vi "write_data.vi"(8 "error in (no error)":errorcluster, 10 "data":T1, 11 "IsotonicRegression in":refnum<class "IsotonicRegression.lvclass">) -> (0 "error out":errorcluster, 3 "IsotonicRegression out":refnum<class "IsotonicRegression.lvclass">)   [LabVIEW 2020, in "IsotonicRegression.lvclass"]
uses:
  IsotonicRegression.lvclass
  Controls/isotonic_regression_data.ctl
  IsotonicRegression.lvclass/IsotonicRegression.ctl
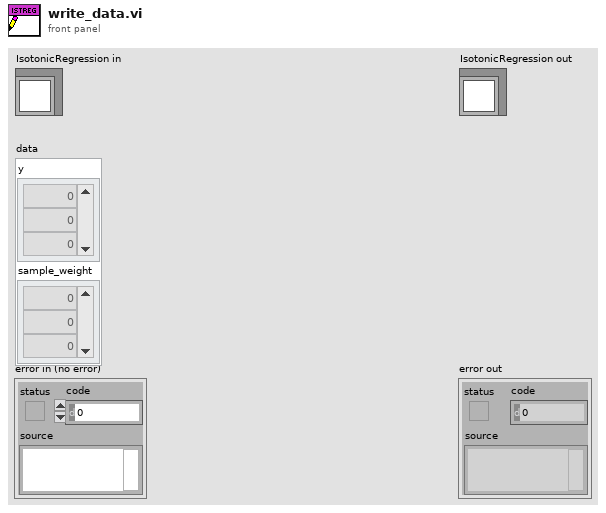
[diagram p1: front panel]
types:
  T1 = typedef "isotonic_regression_data.ctl" = cluster{"y":dbl[], "sample_weight":dbl[]}
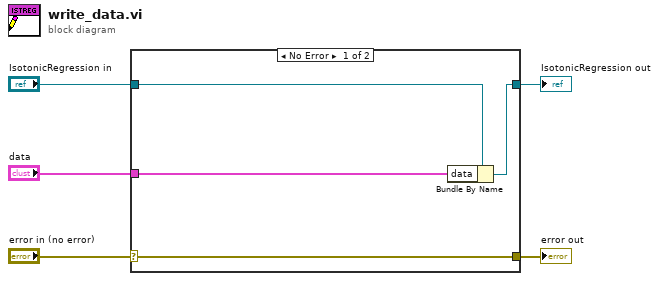
[diagram p0: block diagram]
diagram:
  n1 = case shown="No Error" "error in (no error)" {
    selector: "error in (no error)" -> [w9 w10]
    tunnel: [w9 w10] -> w4
    tunnel: [w7 w11] -> w2
    tunnel: "IsotonicRegression in" -> [w8 w11]
    tunnel: "data" -> [w6 _]
    frame No Error {
      n2 = Bundle By Name(cluster=w8, "data"=w6) -> (w7:refnum<class "IsotonicRegression.lvclass">)
    }
    frame Error {
    }
  }
  "error out" <- w4
  "IsotonicRegression out" <- w2
